vi "test Skipped.vi"(8 "error in (no error)":errorcluster, 11 "Dummy In":refnum<class "Dummy.lvclass">) -> (0 "error out":errorcluster, 3 "Dummy Out":refnum<class "Dummy.lvclass">)   [LabVIEW 2020, in "Dummy.lvclass"]
doc: "Skipped test method"
uses:
  Dummy.lvclass
  C:/git/astemes-lunit/source/Core/LUnit Test Case/LUnit Test Case.lvclass
  API/LUnit Test Case/LUnit Test Case.lvclass/LUnit Test Case.ctl
  API/LUnit Test Case/Private/Append Fail Result.vi
  API/LUnit Test Case/LUnit Test Case.lvclass
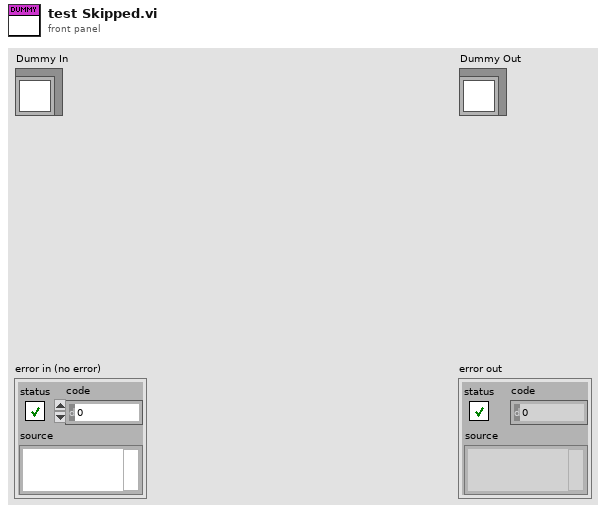
[diagram p1: front panel]
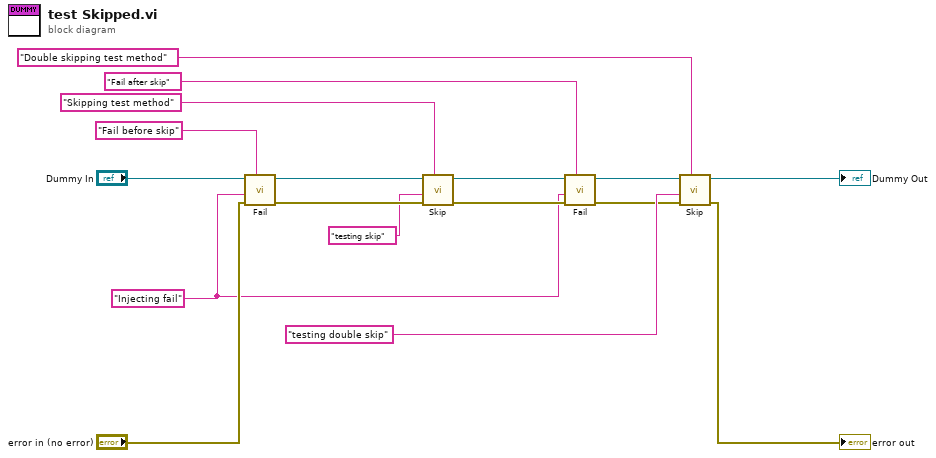
[diagram p0: block diagram]
diagram:
  w7 = "Injecting fail" ("Message")
  n1 = call "Fail.vi"("Description"="Fail before skip", "error in (no error)"="error in (no error)", "Message"=w7, "LUnit Test Case In"="Dummy In") -> ("error out"=w13:errorcluster, "LUnit Test Case Out"=w14:refnum<class "Dummy.lvclass">)  [unwired: 6 in]
  n2 = call "Skip.vi"("Description"="Skipping test method", "error in (no error)"=w13, "Message"="testing skip", "LUnit Test Case In"=w14) -> ("error out"=w16:errorcluster, "LUnit Test Case Out"=w17:refnum<class "Dummy.lvclass">)  [unwired: 6 in]
  n3 = call "Fail.vi"("Description"="Fail after skip", "error in (no error)"=w16, "Message"=w7, "LUnit Test Case In"=w17) -> ("error out"=w2:errorcluster, "LUnit Test Case Out"=w5:refnum<class "Dummy.lvclass">)  [unwired: 6 in]
  n4 = call "Skip.vi"("Description"="Double skipping test method", "error in (no error)"=w2, "Message"="testing double skip", "LUnit Test Case In"=w5) -> ("error out"=→"error out":errorcluster, "LUnit Test Case Out"=→"Dummy Out":refnum<class "Dummy.lvclass">)  [unwired: 6 in]
